vi "CRYASIO Receive Data.vi"(7 "Rcv Idx":i32, 8 "Limit":i32, 10 "Data Length":i32, 11 "Last Remain Buffer":i32[](array[numeric])) -> (0 "Over Load":i32, 2 "Data Out":i32[](array[numeric]), 3 "Remain Data":i32[](array[numeric]))   [LabVIEW 2013]
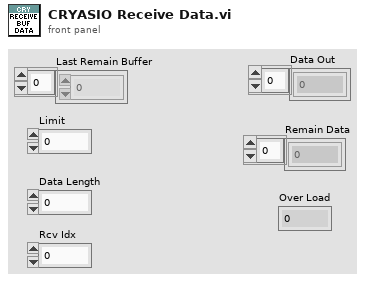
[diagram p1: front panel]
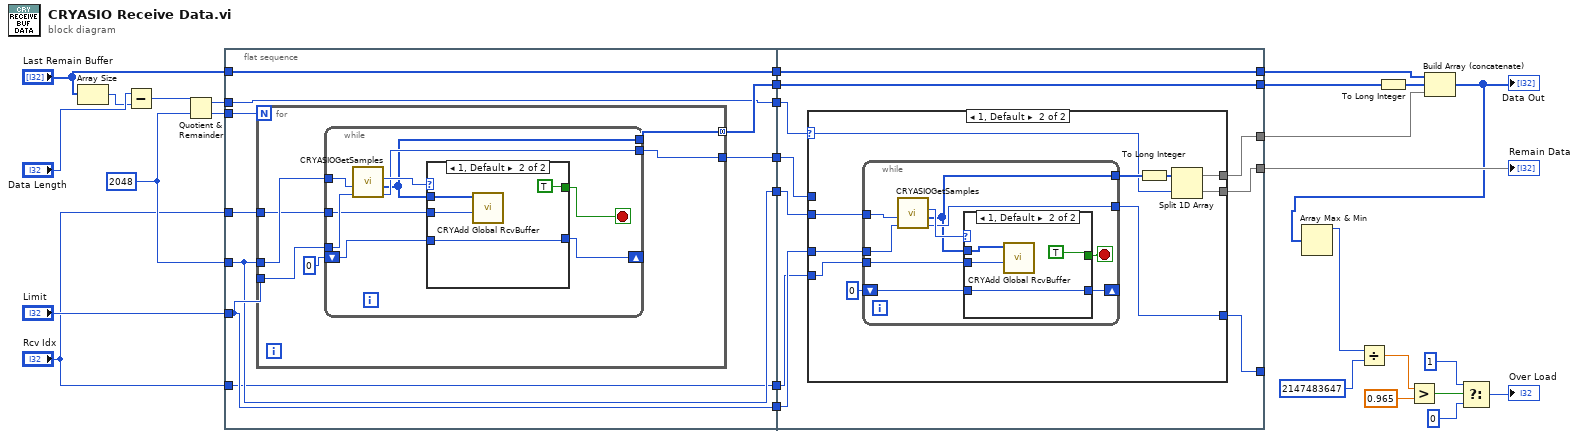
[diagram p0: block diagram]
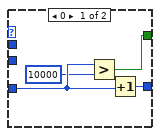
[diagram p2: hidden frame]
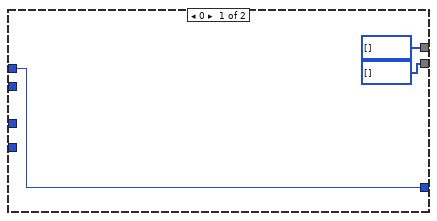
[diagram p3: hidden frame]
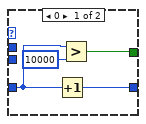
[diagram p4: hidden frame]
diagram:
  w30 = 2048 ("y")
  n1 = Array Size(array="Last Remain Buffer") -> (size(s)=w28:i32)
  n2 = Subtract(x="Data Length", y=w28) -> (x-y=w27:i32)
  n3 = Quotient & Remainder(x=w27, y=w30) -> (x-y*floor(x/y)=w12:i32, floor(x/y)=w26:i32)
  n4 = flat-sequence {
    tunnel: w30 -> [w33]
    tunnel: w26 -> [w39]
    tunnel: "Limit" -> [w34]
    tunnel: [w33] -> w18
    tunnel: [w38] -> w17
    tunnel: [w37] -> w16
    tunnel: [w36] -> w15
    tunnel: "Last Remain Buffer" -> [w36]
    tunnel: w12 -> [w35]
    tunnel: [w35] -> w11
    tunnel: [w34] -> w10
    tunnel: "Rcv Idx" -> [w32]
    tunnel: [w31] -> w7
    tunnel: "Rcv Idx" -> [w31]
    tunnel: [w72] -> w25
    tunnel: w18 -> [w69]
    tunnel: w17 -> [w72]
    tunnel: w16 -> [w65]
    tunnel: w15 -> [w71]
    tunnel: [w71] -> w13
    tunnel: w11 -> [w70]
    tunnel: w10 -> [w64]
    tunnel: [w68] -> w9
    tunnel: [w67] -> w8
    tunnel: [w66] -> _
    tunnel: w7 -> [w63]
    frame #0 {
      n5 = for {
        N: w39 -> [_]
        tunnel: w33 -> [w45]
        tunnel: w34 -> [w43]
        tunnel: [w42] -> w38 mode=concatenating
        tunnel: [w44] -> w37
        tunnel: w32 -> [w41]
        n6 = while {
          tunnel: [w46] -> w42
          tunnel: [w52] -> w44
          tunnel: w45 -> [w51]
          tunnel: w43 -> [w50]
          shift-right: [w48] -> _
          shift-left: 0 ("y") -> [w49]
          tunnel: w41 -> [w47]
          stop <- w53 stop-if-true
          n7 = call "CRYASIOGetSamples.vi"("Limit"=w50, "Data Length"=w51) -> ("Buffer Amount"=w52:i32, "pData"=w46:i32[], "nResult"=w54:u32)  [unwired: 5 in, 1 out]
          n8 = case shown="1, Default" w54 {
            tunnel: [w55 TRUE] -> w53
            tunnel: w49 -> [w57 w61]
            tunnel: [w58 w61] -> w48
            tunnel: w47 -> [_ w60]
            tunnel: w46 -> [_ w59]
            frame 0 {
              n9 = Greater?(x=w57, y=10000) -> (0:w55:bool)
              n10 = Increment(x=w57) -> (x+1=w58:i32)
            }
            frame 1, Default {
              n11 = call "CRYAdd Global RcvBuffer.vi"("Rcv Idx"=w60, "Data"=w59) -> ()  [unwired: 10 in]
            }
          }
        }
      }
    }
    frame #1 {
      n12 = case shown="1, Default" w70 {
        selector: w70 -> [_ w77]
        tunnel: w69 -> [_ w85]
        tunnel: w64 -> [_ w79]
        tunnel: [i32[] [] w83] -> w68
        tunnel: [i32[] [] w82] -> w67
        tunnel: [w73 w81] -> w66
        tunnel: w65 -> [w73 _]
        tunnel: w63 -> [_ w78]
        frame 0 {
        }
        frame 1, Default {
          n13 = while {
            tunnel: [w87] -> w84
            tunnel: [w92] -> w81
            tunnel: w85 -> [w91]
            tunnel: w79 -> [w90]
            shift-right: [w88] -> _
            shift-left: 0 ("y") -> [w89]
            tunnel: w78 -> [w86]
            stop <- w93 stop-if-true
            n14 = call "CRYASIOGetSamples.vi"("Limit"=w90, "Data Length"=w91) -> ("Buffer Amount"=w92:i32, "pData"=w87:i32[], "nResult"=w94:u32)  [unwired: 5 in, 1 out]
            n15 = case shown="1, Default" w94 {
              tunnel: [w95 TRUE] -> w93
              tunnel: w89 -> [w96 w101]
              tunnel: [w98 w101] -> w88
              tunnel: w87 -> [_ w100]
              tunnel: w86 -> [_ w99]
              frame 0 {
                n16 = Increment(x=w96) -> (x+1=w98:i32)
                n17 = Greater?(x=w96, y=10000) -> (0:w95:bool)
              }
              frame 1, Default {
                n18 = call "CRYAdd Global RcvBuffer.vi"("Rcv Idx"=w99, "Data"=w100) -> ()  [unwired: 10 in]
              }
            }
          }
          n19 = To Long Integer(number=w84) -> (32bit integer=w80:i32[])
          n20 = Split 1D Array(array=w80, index=w77) -> (first subarray=w83:i32[], second subarray=w82:i32[])
        }
      }
    }
  }
  n21 = To Long Integer(number=w25) -> (32bit integer=w20:i32[])
  n22 = Build Array (concatenate)(w13, w20, w9) -> (w5:i32[])
  "Data Out" <- w5
  n23 = Array Max & Min(array=w5) -> (max value=w3:i32)  [unwired: 3 out]
  n24 = Divide(x=w3, y=2147483647) -> (x/y=w2:dbl)
  n25 = Greater?(x=w2, y=0.965) -> (0:w24:bool)
  n26 = Select(t=1 ("y"), s=w24, f=0 ("y")) -> (s? t:f=→"Over Load":i32)
  "Remain Data" <- w8
